vi "close.vi"(8 "error in (no error)":errorcluster, 11 "Arduino Uno in":refnum<class "Arduino Uno.lvclass">) -> (0 "error out":errorcluster, 3 "Arduino Uno out":refnum<class "Arduino Uno.lvclass">)   [LabVIEW 2025, in "USB IO.lvlib" / "Arduino Uno.lvclass"]
uses:
  Arduino Uno.lvclass
  Arduino Uno.lvclass/Arduino Uno.ctl
  <vilib>/MakerHub/LINX/LMH-LINX.lvlib
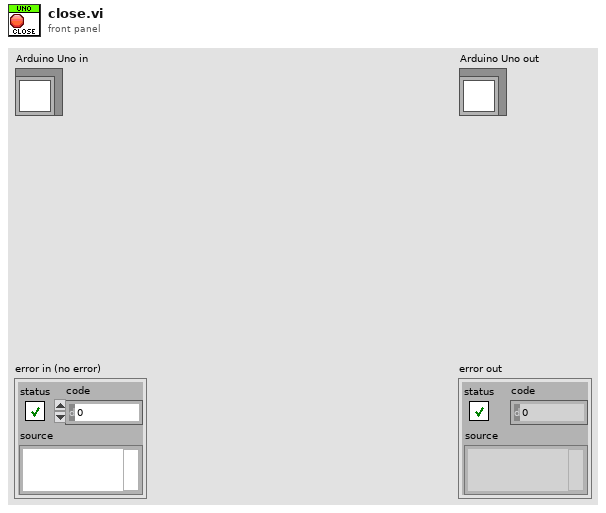
[diagram p1: front panel]
types:
  T1 = typedef "LMH-LINX.lvlib/LINX Ref.ctl" = cluster{"IO":T2, "Interface":T3, "LINX Device Config":T4}
  T2 = typedef "LMH-LINX.lvlib/Platform.ctl" = enum16{"Remote", "Local"}
  T3 = typedef "LMH-LINX.lvlib/Interface.ctl" = enum16{"Serial", "TCP"}
  T4 = typedef "LMH-LINX.lvlib/Device.lvlib/LINX Device Config.ctl" = cluster{"Interface":T3, "COM Port":refnum<visa-resource-name>, "TCP Configuration":T5, "Device Family":u8, "Device ID":u8, "Device Name":string, "TCP Ref":refnum<k5>, "Channels":T6}
  T5 = typedef "LMH-LINX.lvlib/Device.lvlib/TCP Config.ctl" = cluster{"IP Address":string, "Port":u16}
  T6 = typedef "LMH-LINX.lvlib/Channels.ctl" = cluster{"DI":u8[], "DO":u8[], "AI":u8[], "AO":u8[], "PWM":u8[], "QE":u8[], "UART":u8[], "I2C 2":u8[], "SPI":u8[], "CAN":u8[], "Servo":u8[], "AI Ref (V)":dbl, "AI Resolution (Bits)":u8, "AO Ref (V)":dbl, "AO Resolution (Bits)":u8}
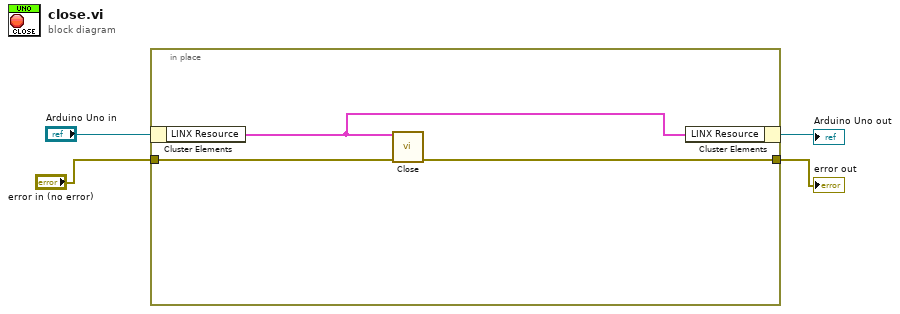
[diagram p0: block diagram]
diagram:
  n1 = in-place {
    in-place-border: [w6] -> w3
    in-place-border: "error in (no error)" -> [w5]
    n2 = in-place-cluster #1("Arduino Uno in") -> ("LINX Resource"=w7:T1)
    n3 = call <vilib>:"Close.vi"("Error In"=w5, "LINX Resource"=w7) -> ("Error Out"=w6:errorcluster)  [unwired: 9 in]
    n4 = in-place-cluster #1("LINX Resource"=w7) -> (→"Arduino Uno out":refnum<class "Arduino Uno.lvclass">)
  }
  "error out" <- w3
